vi "calculate duty cycle.vi"(8 "error in (no error)":errorcluster, 11 "Waveform in":refnum<class "Waveform.lvclass">) -> (0 "error out":errorcluster, 3 "Waveform out":refnum<class "Waveform.lvclass">)   [LabVIEW 2012, in "Waveform.lvclass"]
uses:
  Waveform.lvclass
  Waveform.lvclass/Waveform.ctl
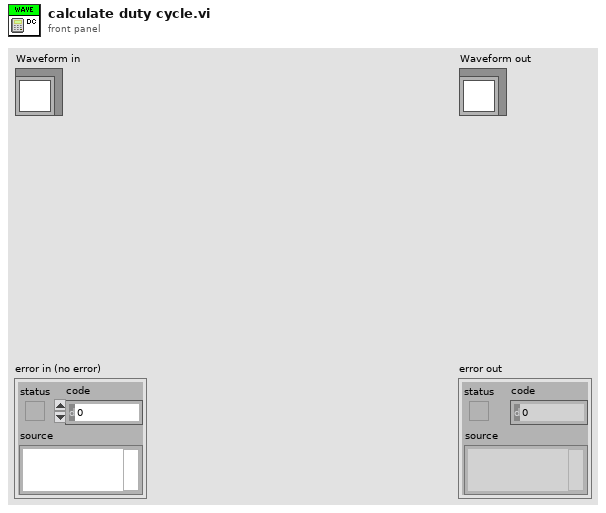
[diagram p1: front panel]
types:
  T1 = cluster{"HSYNC":dbl, "frame_rate":dbl, "y_res":dbl, "line_exp":dbl[unit], "rolling_shutter":dbl[unit]}
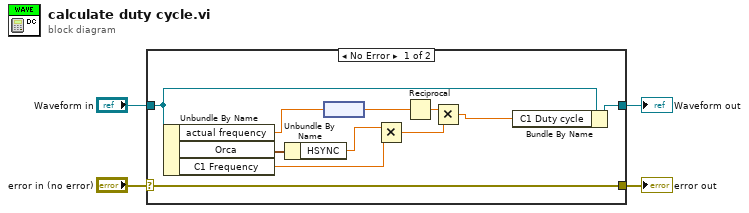
[diagram p0: block diagram]
diagram:
  n1 = case shown="No Error" "error in (no error)" {
    selector: "error in (no error)" -> [w15 w17]
    tunnel: [w15 w17] -> w3
    tunnel: [w10 w16] -> w1
    tunnel: "Waveform in" -> [w11 w16]
    frame No Error {
      n2 = Unbundle By Name(w11) -> ("actual frequency"=w8:dbl[unit], "Orca"=w14:T1, "C1 Frequency"=w9:dbl)
      n3 = Unbundle By Name(w14) -> ("HSYNC"=w13:dbl)
      n4 = node(w8) -> (w6:dbl)
      n5 = Multiply(x=w13, y=w9) -> (x*y=w12:dbl)
      n6 = Reciprocal(x=w6) -> (1/x=w7:dbl)
      n7 = Multiply(x=w7, y=w12) -> (x*y=w5:dbl)
      n8 = Bundle By Name(cluster=w11, "C1 Duty cycle"=w5) -> (w10:refnum<class "Waveform.lvclass">)
    }
    frame Error {
    }
  }
  "error out" <- w3
  "Waveform out" <- w1
